vi "Get Cycle Timing.vi"(11 "Transfer Group Configuration in":refnum<class "Transfer Group Configuration.lvclass">) -> (2 "cycle timing":T1={"priority"=0, "decimation"=1, "offset"=0}, 3 "Transfer Group Configuration out":refnum<class "Transfer Group Configuration.lvclass">)   [LabVIEW 2017, in "Data Sharing Framework Engine.lvlib" / "Transfer Group Configuration.lvclass"]
uses:
  Transfer Group Configuration.lvclass
  DSF Configuration API/1.0.0/Public/Controls/DSF Timing Info.ctl
  Transfer Group Configuration.lvclass/Transfer Group Configuration.ctl
  DSF Configuration API/1.0.0/DSF Configuration API.lvlib
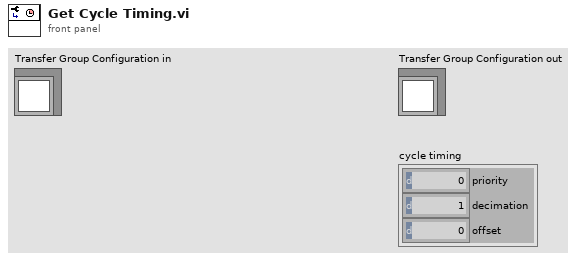
[diagram p1: front panel]
types:
  T1 = typedef "DSF Configuration API.lvlib/DSF Timing Info.ctl" = cluster{"priority":u64, "decimation":u64, "offset":u64}
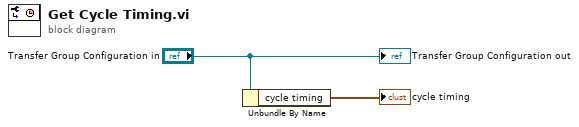
[diagram p0: block diagram]
diagram:
  n1 = Unbundle By Name("Transfer Group Configuration in") -> ("cycle timing"=→"cycle timing":T1)
  "Transfer Group Configuration out" <- "Transfer Group Configuration in"
